vi "BreakLoop.vi"(0 "object in":refnum<class "Application.lvclass">, 5 "error in (no error)":errorcluster) -> (14 "object out":refnum<class "Application.lvclass">, 16 "Abort":bool, 19 "error out":errorcluster)   [LabVIEW 2023, in "Application.lvclass"]
uses:
  Application.lvclass
  Application.lvclass/Application.ctl
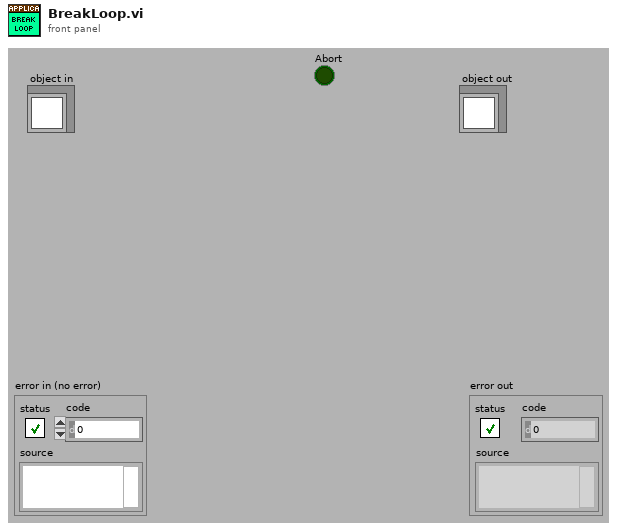
[diagram p1: front panel]
types:
  T1 = cluster{"Message":string, "Message Data":variant}
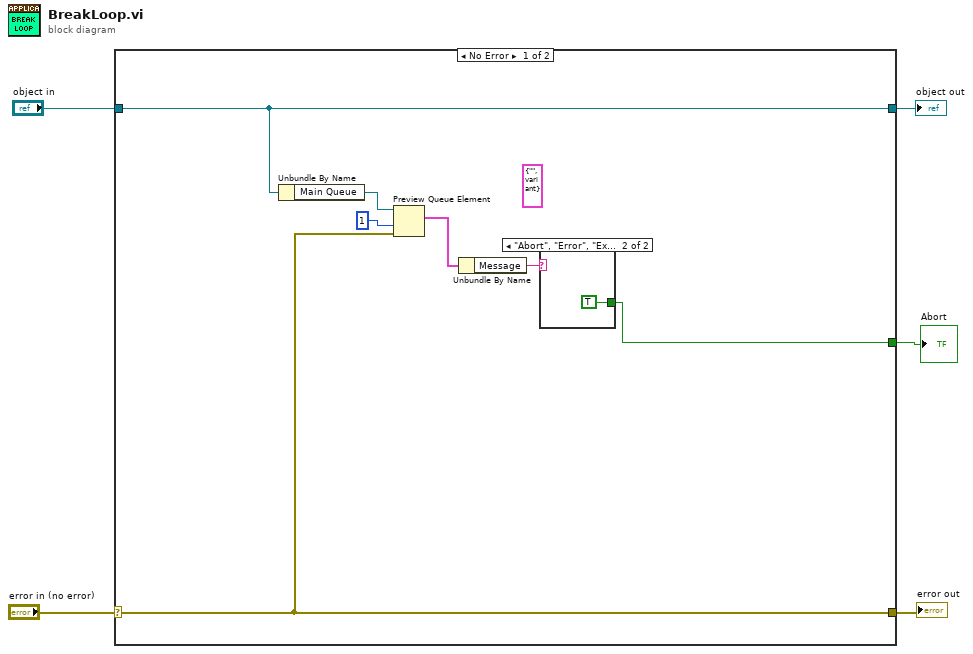
[diagram p0: block diagram]
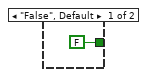
[diagram p2: hidden frame]
diagram:
  n1 = case shown="No Error" "error in (no error)" {
    selector: "error in (no error)" -> [w7 w16]
    tunnel: [w7 w16] -> w4
    tunnel: [w8 w15] -> w2
    tunnel: "object in" -> [w8 w15]
    tunnel: [w6 _] -> w1
    frame No Error {
      (unwired) T1 {"Message"="", "Message Data"=variant} ("element")
      n2 = Unbundle By Name(w8) -> ("Main Queue"=w12:refnum<queue>)
      n3 = Preview Queue Element(queue=w12, timeout in ms (-1)=1, error in (no error)=w7) -> (element=w10:T1)  [unwired: 3 out]
      n4 = Unbundle By Name(w10) -> ("Message"=w9:string)
      n5 = case shown="\"Abort\", \"Error\", \"Exit\"" w9 {
        tunnel: [FALSE TRUE] -> w6
        frame "False", Default {
        }
        frame "Abort", "Error", "Exit" {
        }
      }
    }
    frame Error {
    }
  }
  "error out" <- w4
  "object out" <- w2
  "Abort" <- w1
